vi "Main.vi"() -> ()   [LabVIEW 2012]
panel:
  in  "stop":bool
  in  "Add Mission":bool
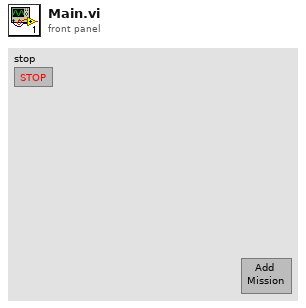
[diagram p1: front panel]
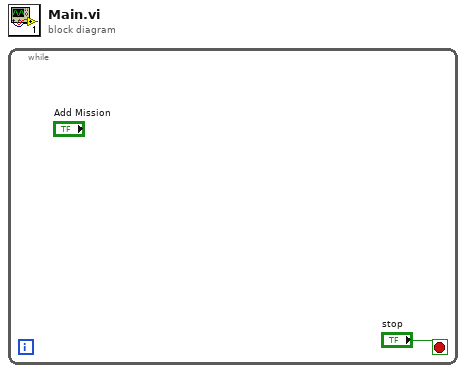
[diagram p0: block diagram]
diagram:
  n1 = while {
    stop <- "stop" stop-if-true
  }
